vi "add_user.vi"(5 "Add Button":bool, 6 "Nom utilisateur":string, 7 "Role":string(combo), 8 "Error out":errorcluster, 9 "Email":string, 10 "Mot de passe":string, 11 "Connection in":refnum<k7>) -> (0 "Error out 2":errorcluster, 3 "Connection Out 2":refnum<k7>)   [LabVIEW 2019]
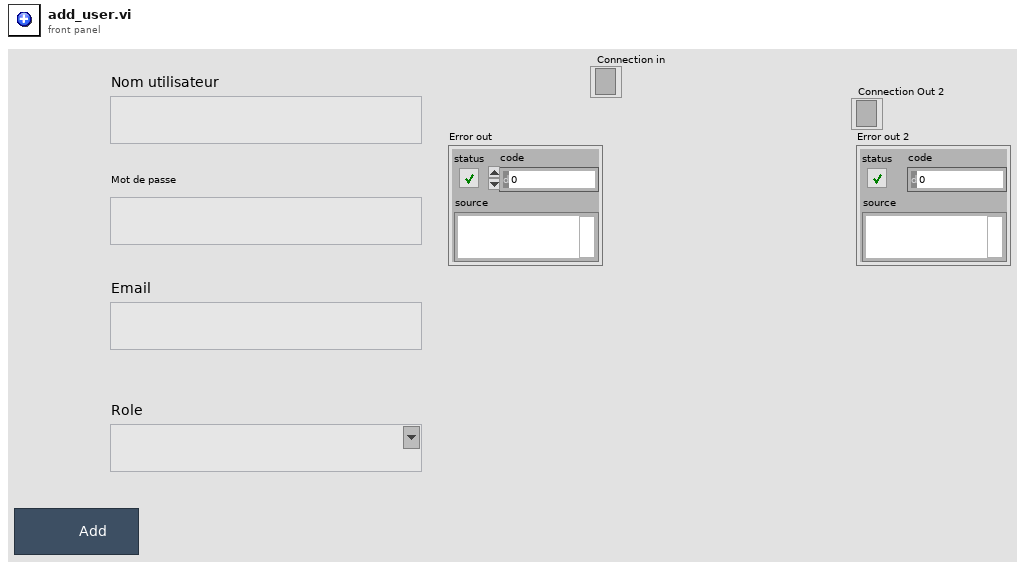
[diagram p1: front panel]
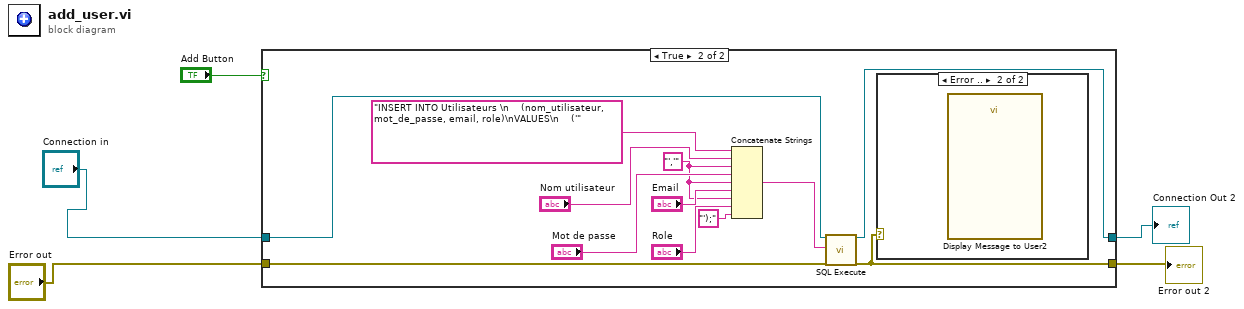
[diagram p0: block diagram]
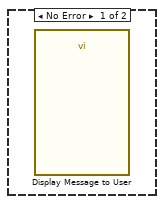
[diagram p3: hidden frame]
diagram:
  n1 = case shown="True" "Add Button" {
    tunnel: "Connection in" -> [w7 w19]
    tunnel: [w6 w9] -> w2
    tunnel: [w7 w18] -> w3
    tunnel: "Error out" -> [w6 w8]
    frame False {
    }
    frame True {
      w12 = "','" ("string")
      n2 = Concatenate Strings("INSERT INTO Utilisateurs \n    (nom_utilisateur, mot_de_passe, email, role)\nVALUES\n    ('" ("SQL Query"), "Nom utilisateur", w12, "Mot de passe", w12, "Email", w12, "Role", "');" ("string")) -> (w17:string)
      n3 = call <vilib>:"SQL Execute.vi"("Connection In"=w19, "SQL Query"=w17, "Error in (no error)"=w8) -> ("Connection Out"=w18:refnum<k7>, "Error out"=w9:errorcluster)  [unwired: 15 in]
      n4 = case shown="Error .." w9 {
        frame No Error {
          n5 = call "Display Message to User"() -> ()  [unwired: 10 in, 2 out]
        }
        frame Error {
          n6 = call "Display Message to User2"() -> ()  [unwired: 10 in, 2 out]
        }
      }
    }
  }
  "Connection Out 2" <- w3
  "Error out 2" <- w2
